vi "Write Outgoing Bytes.vi"(8 "error in (no error)":errorcluster, 9 "timeout (2000 ms)":i32=2000, 10 "Bytes":u8[](array[numeric]) format="%08b", 11 "Connection in":refnum<class "Connection.lvclass">) -> (0 "error out":errorcluster, 3 "Connection out":refnum<class "Connection.lvclass">)   [LabVIEW 2013, in "MQTT_Connection.lvlib" / "Connection.lvclass"]
uses:
  Connection.lvclass
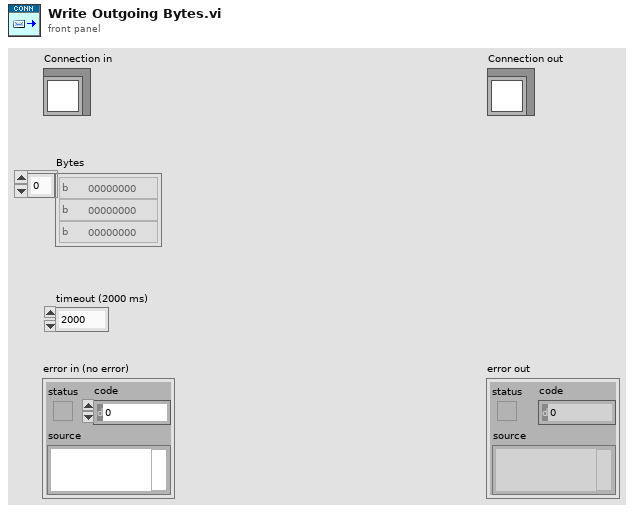
[diagram p1: front panel]
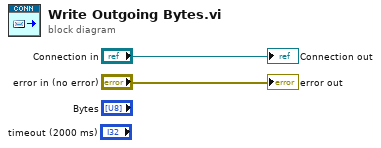
[diagram p0: block diagram]
diagram:
  "error out" <- "error in (no error)"
  "Connection out" <- "Connection in"
